vi "Counts per Second.vi"   [LabVIEW 2013]
types:
  T1 = typedef "WPI_CounterDevRef.ctl" = cluster{"DevStatus":errorcluster, "CntIndex":T2}
  T2 = typedef "FPGA_CounterCtrSystemIndex.ctl" = enum8{"Ctr 0", "Ctr 1", "Ctr 2", "Ctr 3", "Ctr 4", "Ctr 5", "Ctr 6", "Ctr 7", "Invalid"}
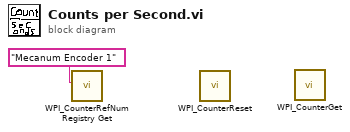
[diagram p0: block diagram]
diagram:
  n1 = call <vilib>:"WPI_CounterRefNum Registry Get.vi"("refnum name"="Mecanum Encoder 1") -> ("CounterDevRef"=w4:T1)  [unwired: 9 in, 1 out]
  n2 = call <vilib>:"WPI_CounterReset.vi"() -> ("CounterDevRef out"=w1:T1, "CounterDevRef in"=w2:T1)  [unwired: 9 in, 1 out]
  n3 = call <vilib>:"WPI_CounterGet.vi"() -> ()  [unwired: 6 in, 6 out]
